vi "Wait On Launched Notifier.vi"(8 "error in (no error)":errorcluster, 10 "Launch Timeout [ms]":i32, 11 "Actor in":refnum<class "Actor.lvclass">) -> (0 "error out":errorcluster, 2 "Launch Time":timestamp, 3 "Actor out":refnum<class "Actor.lvclass">)   [LabVIEW 2015, in "Actor.lvclass"]
uses:
  Actor.lvclass
  Actor.lvclass/Actor.ctl
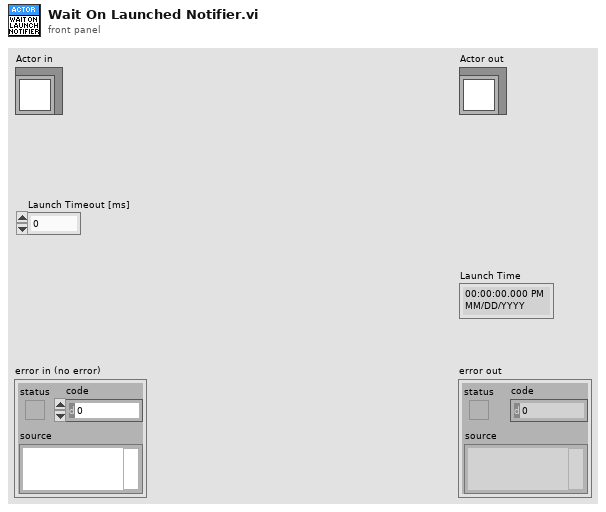
[diagram p1: front panel]
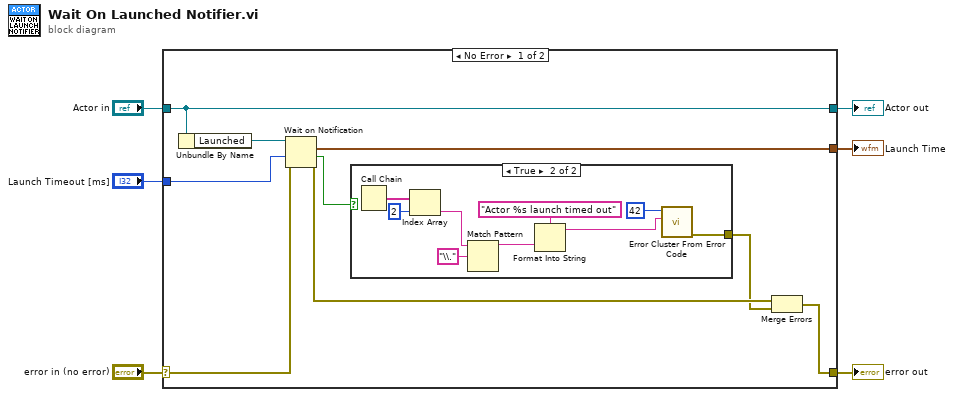
[diagram p0: block diagram]
diagram:
  n1 = case shown="No Error" "error in (no error)" {
    selector: "error in (no error)" -> [w14 w26]
    tunnel: [w8 w26] -> w5
    tunnel: [w15 w25] -> w3
    tunnel: "Actor in" -> [w15 w25]
    tunnel: "Launch Timeout [ms]" -> [w12 _]
    tunnel: [w11 _] -> w1
    frame No Error {
      n2 = Unbundle By Name(w15) -> ("Launched"=w13:refnum<notifier>)
      n3 = Wait on Notification(notifier=w13, timeout in ms (-1)=w12, error in (no error)=w14) -> (notification=w11:timestamp, timed out?=w7:bool, error out=w10:errorcluster)  [unwired: 1 in, 1 out]
      n4 = case shown="True" w7 {
        tunnel: [_ w23] -> w9
        frame False {
        }
        frame True {
          n5 = Call Chain() -> (call chain=w22:string[])
          n6 = Index Array(array=w22, index=2) -> (element=w17:string)
          n7 = Match Pattern(string=w17, regular expression="\\.") -> (before substring=w16:string)  [unwired: 1 in, 3 out]
          n8 = Format Into String(format string="Actor %s launch timed out", w16) -> (resulting string=w19:string)  [unwired: 2 in, 1 out]
          n9 = call <vilib>:"Error Cluster From Error Code.vi"("error message (\"\")"=w19, "error code (0)"=42) -> ("error out"=w23:errorcluster)  [unwired: 7 in]
        }
      }
      n10 = Merge Errors(w10, w9) -> (w8:errorcluster)
    }
    frame Error {
    }
  }
  "error out" <- w5
  "Actor out" <- w3
  "Launch Time" <- w1
